vi "Aimbot.vi"(1 "Firing Data":T1={"error"={"status"=FALSE, "code"=0, "source"=""}, "AngleMotorRefnum"={"DeviceStatus"={"status"=FALSE, "code"=0, "source"=""}, "Type"=enum."PWM", "PWM"={"PWM Channel"=enum."PWM 1", "DeadBand"={"Name"="", "maxPositivePwm"=0, "minPositivePwm"=0, "centerPwm"=0, "maxNegativePwm"=0, "minNegativePwm"=0, "angularRange"=0}}, "CAN"={"Device Number"=0, "Control Mode"=enum."Percent VBus", "Semaphore"=refnum, "Max Vout"=12.0, "TalonSRX Control Mode"=enum."Percent VBus"}, "Invert"=FALSE}, "LeftWheelRefnum"={"DeviceStatus"={"status"=FALSE, "code"=0, "source"=""}, "Type"=enum."PWM", "PWM"={"PWM Channel"=enum."Invalid", "DeadBand"={"Name"="", "maxPositivePwm"=0, "minPositivePwm"=0, "centerPwm"=0, "maxNegativePwm"=0, "minNegativePwm"=0, "angularRange"=0}}, "CAN"={"Device Number"=0, "Control Mode"=enum."Percent VBus", "Semaphore"=refnum, "Max Vout"=12.0, "TalonSRX Control Mode"=enum."Percent VBus"}, "Invert"=FALSE}, "RightWheelRefnum"={"DeviceStatus"={"status"=FALSE, "code"=0, "source"=""}, "Type"=enum."PWM", "PWM"={"PWM Channel"=enum."Invalid", "DeadBand"={"Name"="", "maxPositivePwm"=0, "minPositivePwm"=0, "centerPwm"=0, "maxNegativePwm"=0, "minNegativePwm"=0, "angularRange"=0}}, "CAN"={"Device Number"=0, "Control Mode"=enum."Percent VBus", "Semaphore"=refnum, "Max Vout"=12.0, "TalonSRX Control Mode"=enum."Percent VBus"}, "Invert"=FALSE}, "PushSolenoidRefnum"={"DevStatus"={"status"=FALSE, "code"=0, "source"=""}, "Pneumatics Control Module"=0, "Forward Solenoid Channel"=enum."Invalid", "Reverse Solenoid Channel"=enum."Invalid"}, "AngleMotorPosition(t)"=0.0, "LaunchSpeed(t/100ms)"=0.0, "CollectSpeed(t/100ms)"=0.0, "AngleThreshold"=0.0, "ShotDuration(10ms)"=0}, 2 "Range":dbl) -> (0 "Firing Data out":T1={"error"={"status"=FALSE, "code"=0, "source"=""}, "AngleMotorRefnum"={"DeviceStatus"={"status"=FALSE, "code"=0, "source"=""}, "Type"=enum."PWM", "PWM"={"PWM Channel"=enum."PWM 1", "DeadBand"={"Name"="", "maxPositivePwm"=0, "minPositivePwm"=0, "centerPwm"=0, "maxNegativePwm"=0, "minNegativePwm"=0, "angularRange"=0}}, "CAN"={"Device Number"=0, "Control Mode"=enum."Percent VBus", "Semaphore"=refnum, "Max Vout"=12.0, "TalonSRX Control Mode"=enum."Percent VBus"}, "Invert"=FALSE}, "LeftWheelRefnum"={"DeviceStatus"={"status"=FALSE, "code"=0, "source"=""}, "Type"=enum."PWM", "PWM"={"PWM Channel"=enum."Invalid", "DeadBand"={"Name"="", "maxPositivePwm"=0, "minPositivePwm"=0, "centerPwm"=0, "maxNegativePwm"=0, "minNegativePwm"=0, "angularRange"=0}}, "CAN"={"Device Number"=0, "Control Mode"=enum."Percent VBus", "Semaphore"=refnum, "Max Vout"=12.0, "TalonSRX Control Mode"=enum."Percent VBus"}, "Invert"=FALSE}, "RightWheelRefnum"={"DeviceStatus"={"status"=FALSE, "code"=0, "source"=""}, "Type"=enum."PWM", "PWM"={"PWM Channel"=enum."Invalid", "DeadBand"={"Name"="", "maxPositivePwm"=0, "minPositivePwm"=0, "centerPwm"=0, "maxNegativePwm"=0, "minNegativePwm"=0, "angularRange"=0}}, "CAN"={"Device Number"=0, "Control Mode"=enum."Percent VBus", "Semaphore"=refnum, "Max Vout"=12.0, "TalonSRX Control Mode"=enum."Percent VBus"}, "Invert"=FALSE}, "PushSolenoidRefnum"={"DevStatus"={"status"=FALSE, "code"=0, "source"=""}, "Pneumatics Control Module"=0, "Forward Solenoid Channel"=enum."Invalid", "Reverse Solenoid Channel"=enum."Invalid"}, "AngleMotorPosition(t)"=0.0, "LaunchSpeed(t/100ms)"=0.0, "CollectSpeed(t/100ms)"=0.0, "AngleThreshold"=0.0, "ShotDuration(10ms)"=0})   [LabVIEW 2015]
doc: "Aims and fires according to vision."
uses:
  Bundle.ctl
  <vilib>/Rock Robotics/WPI/MotorControl/WPI_MotorControlDeviceRef.ctl
  <vilib>/Rock Robotics/WPI/MotorControl/WPI_MotorControlType.ctl
  <vilib>/Rock Robotics/SystemInterfaces/DIO/FPGA_DIOPWMChannel.ctl
  <vilib>/Rock Robotics/WPI/PWM/WPI_PWMDeadband.ctl
  <vilib>/Rock Robotics/WPI/CAN/Jaguar/SubVIs/WPI_CANJaguar_ControlMode.ctl
  <vilib>/Rock Robotics/WPI/CAN/TalonSRX/WPI_CANTalonSRX_APIControlMode.ctl
  <vilib>/Rock Robotics/WPI/Solenoid/WPI_SolenoidDevRef.ctl
  <vilib>/Rock Robotics/WPI/Solenoid/WPI_SolenoidChannel.ctl
  <vilib>/Rock Robotics/WPI/Solenoid/WPI_SolenoidValue.ctl
  Robot Global Data.vi
  <vilib>/Rock Robotics/WPI/Solenoid/WPI_SolenoidSetEnum.vi
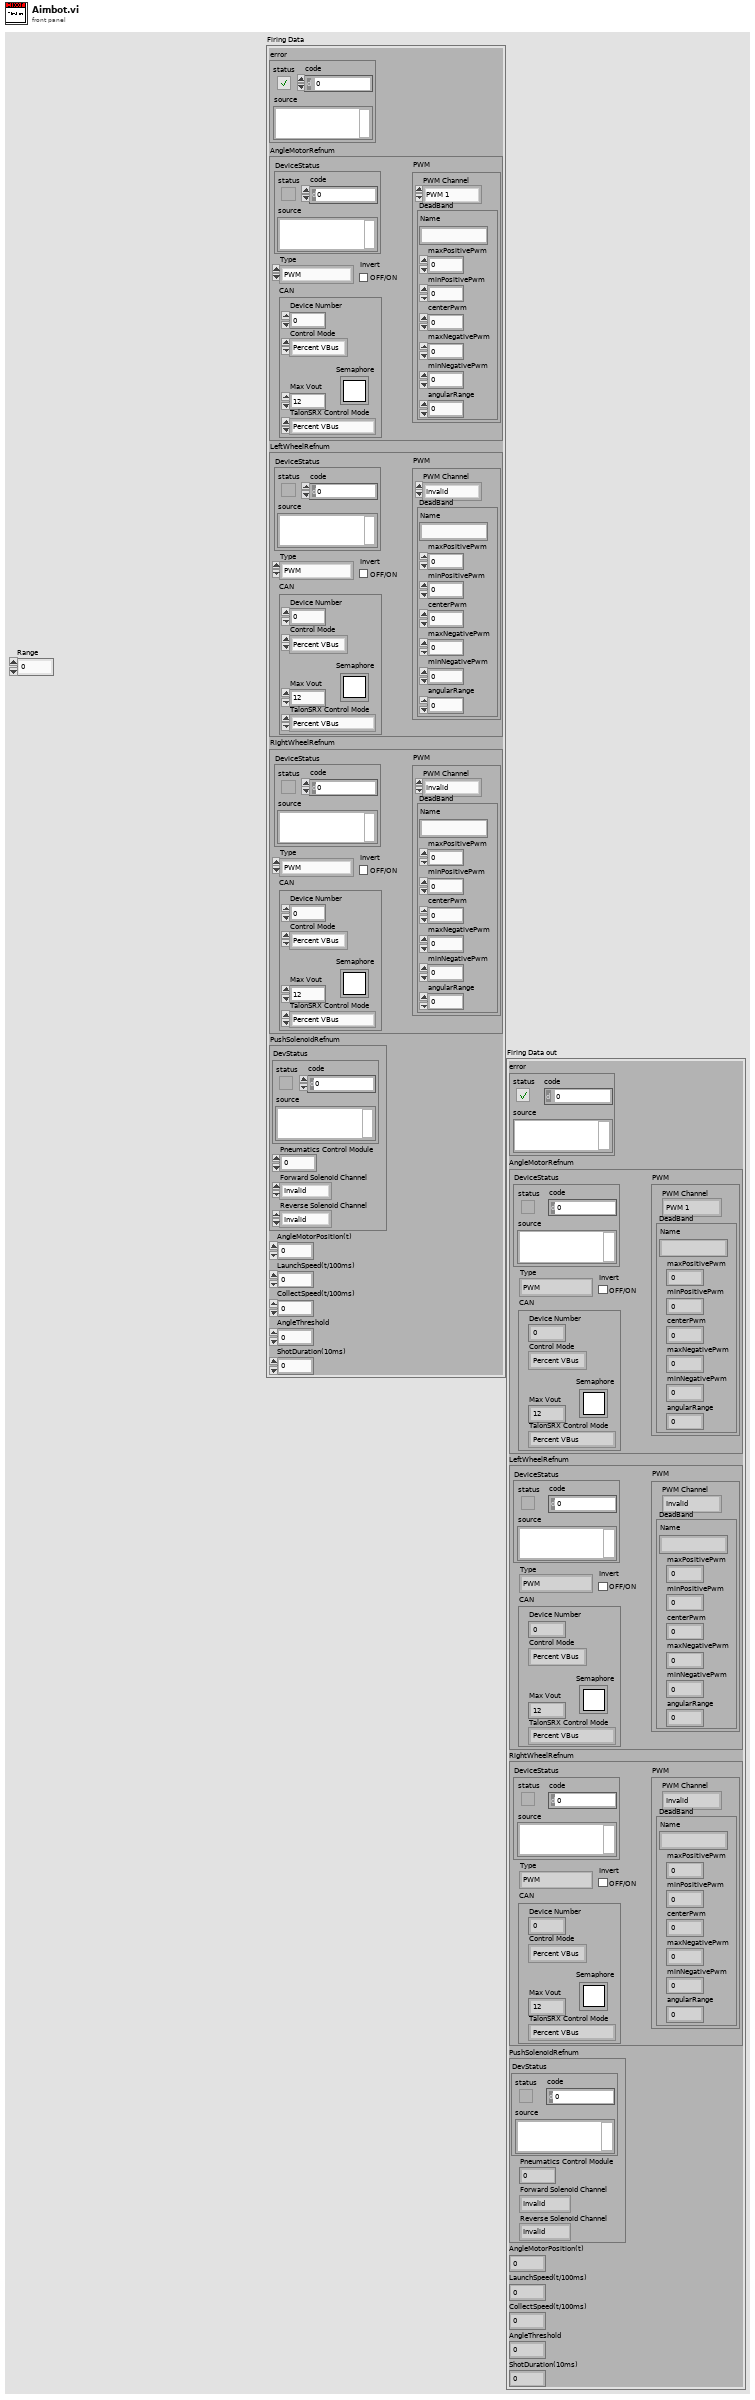
[diagram p1: front panel]
types:
  T1 = typedef "Bundle.ctl" = cluster{"error":errorcluster, "AngleMotorRefnum":T2, "LeftWheelRefnum":T2, "RightWheelRefnum":T2, "PushSolenoidRefnum":T9, "AngleMotorPosition(t)":dbl, "LaunchSpeed(t/100ms)":dbl, "CollectSpeed(t/100ms)":dbl, "AngleThreshold":dbl, "ShotDuration(10ms)":i32}
  T2 = typedef "WPI_MotorControlDeviceRef.ctl" = cluster{"DeviceStatus":errorcluster, "Type":T3, "PWM":cluster{"PWM Channel":T4, "DeadBand":T5}, "CAN":cluster{"Device Number":u8, "Control Mode":T6, "Semaphore":T7, "Max Vout":dbl, "TalonSRX Control Mode":T8}, "Invert":bool}
  T3 = typedef "WPI_MotorControlType.ctl" = enum16{"PWM", "CAN", "CANTalonSRX"}
  T4 = typedef "FPGA_DIOPWMChannel.ctl" = enum8{"PWM 0", "PWM 1", "PWM 2", "PWM 3", "PWM 4", "PWM 5", "PWM 6", "PWM 7", "PWM 8", "PWM 9", "PWM MXP 0", "PWM MXP 1", "PWM MXP 2", "PWM MXP 3", "PWM MXP 4", "PWM MXP 5", "PWM MXP 6", "PWM MXP 7", "PWM MXP 8", "PWM MXP 9", "Invalid"}
  T5 = typedef "WPI_PWMDeadband.ctl" = cluster{"Name":string, "maxPositivePwm":i32, "minPositivePwm":i32, "centerPwm":i32, "maxNegativePwm":i32, "minNegativePwm":i32, "angularRange":u16}
  T6 = typedef "WPI_CANJaguar_ControlMode.ctl" = enum8{"Percent VBus", "Current", "Speed", "Position", "Voltage"}
  T7 = typedef "Semaphore RefNum" = refnum<k1>
  T8 = typedef "WPI_CANTalonSRX_APIControlMode.ctl" = enum8{"Percent VBus", "Speed", "Position", "Slave", "Unchanged / Invalid", "Voltage Compensation", "Current", "Motion Profile"}
  T9 = typedef "WPI_SolenoidDevRef.ctl" = cluster{"DevStatus":errorcluster, "Pneumatics Control Module":u8, "Forward Solenoid Channel":T10, "Reverse Solenoid Channel":T10}
  T10 = typedef "WPI_SolenoidChannel.ctl" = enum8{"Solenoid 0", "Solenoid 1", "Solenoid 2", "Solenoid 3", "Solenoid 4", "Solenoid 5", "Solenoid 6", "Solenoid 7", "Invalid"}
  T11 = cluster{"Firing Angle":dbl, "Max Angle?":bool, "Min Angle?":bool}
  T12 = typedef "WPI_SolenoidValue.ctl" = enum16{"Off", "On", "Forward", "Reverse"}
  T13 = typedef "WPI_CANTalonSRX_GlobalStatus.ctl" = cluster{"Applied Throttle":dbl, "Module Enabled":bool, "CAN Error":errorcluster, "Closed Loop Error":dbl, "Forward Limit Switch Closed":bool, "Reverse Limit Switch Closed":bool, "Sensor Position":dbl, "Sensor Velocity":dbl, "Current":dbl, "Sticky Fault - Over Temp":bool, "Sticky Fault - Under Voltage":bool, "Sticky Fault - Forward Limit":bool, "Sticky Fault - Reverse Limit":bool, "Sticky Fault - Forward Soft Limit":bool, "Sticky Fault - Reverse Soft Limit":bool, "Brake is Enabled":bool, "Encoder Position":dbl, "Encoder Velocity":dbl, "Encoder Index Count":dbl, "Encoder A Pin State":bool, "Encoder B Pin State":bool, "Encoder Index Pin State":bool, "Analog In":dbl, "Analog In Velocity":dbl, "Temperature (C)":dbl, "Battery Voltage":dbl, "Control 5 Is Supported":bool, "Current Profile Slot Select":dbl, "Pos Div 8":bool, "Vel Div 4":bool, "Pulse Width Position":i32, "Pulse Width Velocity":i32, "Pulse Width Rise To Rise (us)":i32, "Pulse Width Rise To Fall (us)":i32, "Mot Prof Active Is Under Run":bool, "Mot Prof Active Has Under Run":bool, "Mot Prof Active Is Last":bool, "Mot Prof Active Velocity Only":bool, "Mot Prof Active Is Valid":bool, "Mot Prof Buffer Is Full":bool, "Mot Prof Active Profile Slot Select":i32, "Mot Prof NextID":i32, "Mot Prof Count":i32, "Mot Prof Active Velocity":dbl, "Mot Prof Active Position":dbl, "Mot Prof Output Enable":i32}
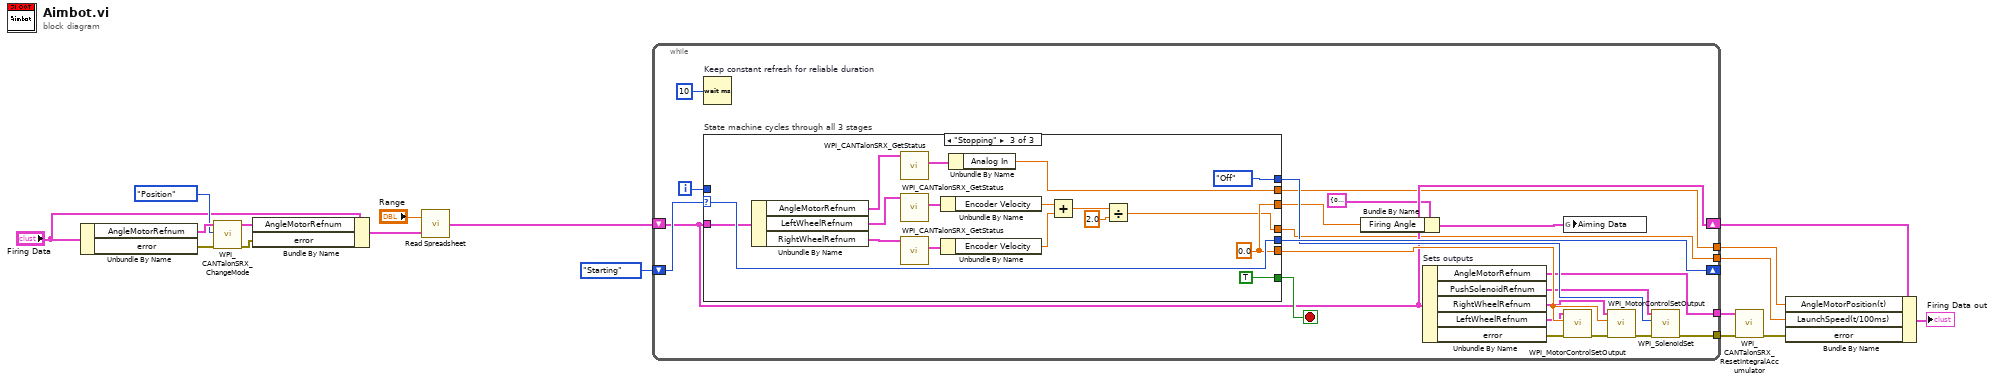
[diagram p0: block diagram]
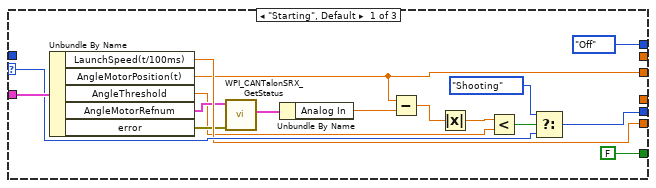
[diagram p2: hidden frame]
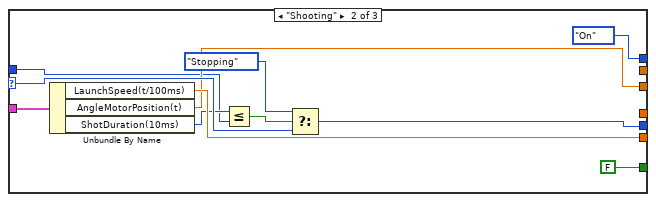
[diagram p3: hidden frame]
diagram:
  n1 = Unbundle By Name("Firing Data") -> ("AngleMotorRefnum"=w7:T2, "error"=w5:errorcluster)
  n2 = call <vilib>:"WPI_CANTalonSRX_ChangeMode.vi"("error in (no error)"=w5, "Control Mode"=WPI_CANTalonSRX_APIControlMode."Position", "CAN Talon SRX Ref"=w7) -> ("error out"=w3:errorcluster, "CAN Talon SRX Ref"=w4:T2)  [unwired: 7 in]
  n3 = Bundle By Name(cluster="Firing Data", "AngleMotorRefnum"=w4, "error"=w3) -> (w1:T1)
  n4 = call "Read Spreadsheet.vi"("Firing Data"=w1, "Range"="Range") -> ("Firing Data"=w15:T1)
  n5 = while {
    shift-right: [w35] -> _
    shift-left: enum16{"Starting", "Shooting", "Stopping"}."Starting" -> [w38]
    shift-right: [w25] -> w12
    shift-left: w15 -> [w25]
    tunnel: [w22] -> w14
    tunnel: [w24] -> w9
    tunnel: [w23] -> w10
    tunnel: [w21] -> w8
    i -> [w36]
    stop <- w32 stop-if-true
    n6 = Wait (ms) "Keep constant refresh for reliable duration"(milliseconds to wait=u32 10) -> ()  [unwired: 1 out]
    n7 = case "State machine cycles through all 3 stages" shown="\"Stopping\"" w38 {
      selector: w38 -> [w53 w64 w82]
      tunnel: w36 -> [_ w56 _]
      tunnel: w25 -> [w54 w65 w77]
      tunnel: [w52 w63 w82] -> w35
      tunnel: [w48 w59 w81] -> w34
      tunnel: [w44 w58 w81] -> w18
      tunnel: [FALSE FALSE TRUE] -> w32
      tunnel: [WPI_SolenoidValue."Off" ("Value") WPI_SolenoidValue."On" ("Value") WPI_SolenoidValue."Off" ("Value")] -> w31
      tunnel: [_ _ w67] -> w24
      tunnel: [_ _ w66] -> w23
      frame "Starting", Default {
        n8 = Unbundle By Name(w54) -> ("LaunchSpeed(t/100ms)"=w48:dbl, "AngleMotorPosition(t)"=w44:dbl, "AngleThreshold"=w39:dbl, "AngleMotorRefnum"=w46:T2, "error"=w45:errorcluster)
        n9 = call <vilib>:"WPI_CANTalonSRX_GetStatus.vi"("error in (no error)"=w45, "CAN Talon SRX Ref"=w46) -> ("Talon SRX Status"=w47:T13)  [unwired: 7 in, 2 out]
        n10 = Unbundle By Name(w47) -> ("Analog In"=w43:dbl)
        n11 = Subtract(x=w44, y=w43) -> (x-y=w42:dbl)
        n12 = Absolute Value(x=w42) -> (abs(x)=w41:dbl)
        n13 = Less?(x=w41, y=w39) -> (x < y?=w40:bool)
        n14 = Select(t=enum16{"Starting", "Shooting", "Stopping"}."Shooting", s=w40, f=w53) -> (s? t:f=w52:enum16{"Starting", "Shooting", "Stopping"})
      }
      frame "Shooting" {
        n15 = Unbundle By Name(w65) -> ("LaunchSpeed(t/100ms)"=w59:dbl, "AngleMotorPosition(t)"=w58:dbl, "ShotDuration(10ms)"=w57:i32)
        n16 = Less Or Equal?(x=w57, y=w56) -> (x <= y?=w55:bool)
        n17 = Select(t=enum16{"Starting", "Shooting", "Stopping"}."Stopping", s=w55, f=w64) -> (s? t:f=w63:enum16{"Starting", "Shooting", "Stopping"})
      }
      frame "Stopping" {
        w81 = 0.0 ("AngleMotorT")
        n18 = Unbundle By Name(w77) -> ("AngleMotorRefnum"=w76:T2, "LeftWheelRefnum"=w73:T2, "RightWheelRefnum"=w72:T2)
        n19 = call <vilib>:"WPI_CANTalonSRX_GetStatus.vi"("CAN Talon SRX Ref"=w76) -> ("Talon SRX Status"=w78:T13)  [unwired: 8 in, 2 out]
        n20 = call <vilib>:"WPI_CANTalonSRX_GetStatus.vi"("CAN Talon SRX Ref"=w73) -> ("Talon SRX Status"=w75:T13)  [unwired: 8 in, 2 out]
        n21 = call <vilib>:"WPI_CANTalonSRX_GetStatus.vi"("CAN Talon SRX Ref"=w72) -> ("Talon SRX Status"=w74:T13)  [unwired: 8 in, 2 out]
        n22 = Unbundle By Name(w75) -> ("Encoder Velocity"=w69:dbl)
        n23 = Unbundle By Name(w74) -> ("Encoder Velocity"=w68:dbl)
        n24 = Unbundle By Name(w78) -> ("Analog In"=w66:dbl)
        n25 = Add(x=w69, y=w68) -> (x+y=w70:dbl)
        n26 = Divide(x=w70, y=2.0) -> (x/y=w67:dbl)
      }
    }
    n27 = Bundle By Name(cluster=T11 {"Firing Angle"=0.0, "Max Angle?"=FALSE, "Min Angle?"=FALSE} ("Aiming Data"), "Firing Angle"=w18) -> (w19:T11)
    n28 = Unbundle By Name "Sets outputs"(w25) -> ("AngleMotorRefnum"=w21:T2, "PushSolenoidRefnum"=w28:T9, "RightWheelRefnum"=w27:T2, "LeftWheelRefnum"=w26:T2, "error"=w29:errorcluster)
    n29 = global write "Robot Global Data.vi" "Aiming Data"(w19) -> ()
    n30 = call <vilib>:"WPI_MotorControlSetOutput.vi"("error in (no error)"=w29, "Output"=w34, "MotorControlDevRef"=w26) -> ("error out"=w33:errorcluster)  [unwired: 6 in, 2 out]
    n31 = call <vilib>:"WPI_MotorControlSetOutput.vi"("error in (no error)"=w33, "Output"=w34, "MotorControlDevRef"=w27) -> ("error out"=w30:errorcluster)  [unwired: 6 in, 2 out]
    n32 = call-poly <vilib>:"WPI_SolenoidSet.vi"("error in (no error)"=w30, "Value"=w31, "SolenoidDevRef"=w28) -> ("error out"=w22:errorcluster)  [unwired: 7 in, 1 out]
  }
  n33 = call <vilib>:"WPI_CANTalonSRX_ResetIntegralAccumulator.vi"("error in (no error)"=w14, "CAN Talon SRX Ref"=w8) -> ("error out"=w13:errorcluster)  [unwired: 8 in, 1 out]
  n34 = Bundle By Name(cluster=w12, "AngleMotorPosition(t)"=w10, "LaunchSpeed(t/100ms)"=w9, "error"=w13) -> (→"Firing Data out":T1)
